vi "Remove State Frame.vi"(8 "error in (no error)":errorcluster, 10 "element":string, 11 "CSM-Helper in":refnum<class "CSM-Helper.lvclass">) -> (0 "error out":errorcluster, 3 "CSM-Helper out":refnum<class "CSM-Helper.lvclass">)   [LabVIEW 2017, in "CSM-Helper.lvclass"]
doc: "### Remove State Frame.vi\n\n-- <b>Controls</b> --\n- <b>element</b>:\n- <b>CSM-Helper in</b>: CSMHelper input\n\n-- <b>Indicators</b> --\n- <b>CSM-Helper out</b>: CSMHelper output"
uses:
  CSM-Helper.lvclass
  CSM-Helper.lvclass/CSM-Helper.ctl
  Properties/Read Case Structure Ref.vi
  Get CaseFrame Index By CaseName.vi
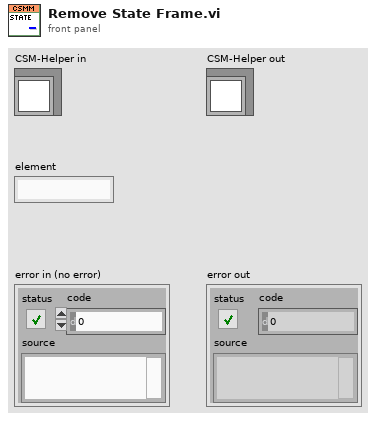
[diagram p1: front panel]
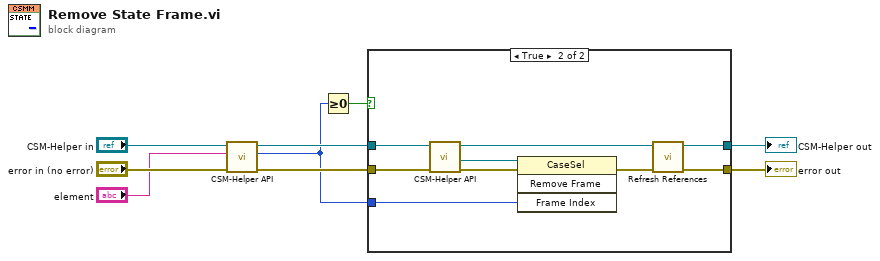
[diagram p0: block diagram]
diagram:
  n1 = call-poly "CSM-Helper API.vi"("error in (no error)"="error in (no error)", "CASE"="element", "CSM-Helper in"="CSM-Helper in") -> ("error out"=w3:errorcluster, "index"=w2:i32, "CSM-Helper out"=w8:refnum<class "CSM-Helper.lvclass">)  [unwired: 5 in, 1 out]
  n2 = Greater Or Equal To 0?(x=w2) -> (x >= 0?=w1:bool)
  n3 = case shown="True" w1 {
    tunnel: w8 -> [w10 w20]
    tunnel: [w11 w19] -> w7
    tunnel: [w10 w18] -> w6
    tunnel: w3 -> [w11 w16]
    tunnel: w2 -> [_ w12]
    frame False {
    }
    frame True {
      n4 = call-poly "CSM-Helper API.vi"("error in (no error)"=w16, "CSM-Helper in"=w20) -> ("error out"=w15:errorcluster, "Case Structure"=w13:refnum<vi>, "CSM-Helper out"=w17:refnum<class "CSM-Helper.lvclass">)  [unwired: 7 in]
      n5 = invoke class="CaseSel" method="Remove Frame"(reference=w13, error in=w15, "Frame Index"=w12) -> (error out=w14:errorcluster)  [unwired: 1 in, 3 out]
      n6 = call "Refresh References.vi"("error in (no error)"=w14, "CSM-Helper in"=w17) -> ("error out"=w19:errorcluster, "CSM-Helper out"=w18:refnum<class "CSM-Helper.lvclass">)  [unwired: 8 in]
    }
  }
  "error out" <- w7
  "CSM-Helper out" <- w6
